vi "Configure CAN Read Gen.vi"(8 "error in":errorcluster, 11 "measurement configuration":T1 {"Baudrate" format="%x"; "FD Baudrate" format="%x"}) -> (0 "error out":errorcluster, 3 "XNET Read":refnum<k21>)   [LabVIEW 2025]
uses:
  <resource>/objmgr/xnet.rc
  <vilib>/xnet/xnet.llb/XNET Create Session (Frame Input Stream).vi
  can-lin/CAN-LIN Raw Bus Capture UI/Toggle.ctl
  can-lin/CAN-LIN Raw Bus Capture/Measurement Configuration.ctl
  can-lin/CAN-LIN Raw Bus Capture/CAN-LIN Raw Bus Capture.lvclass
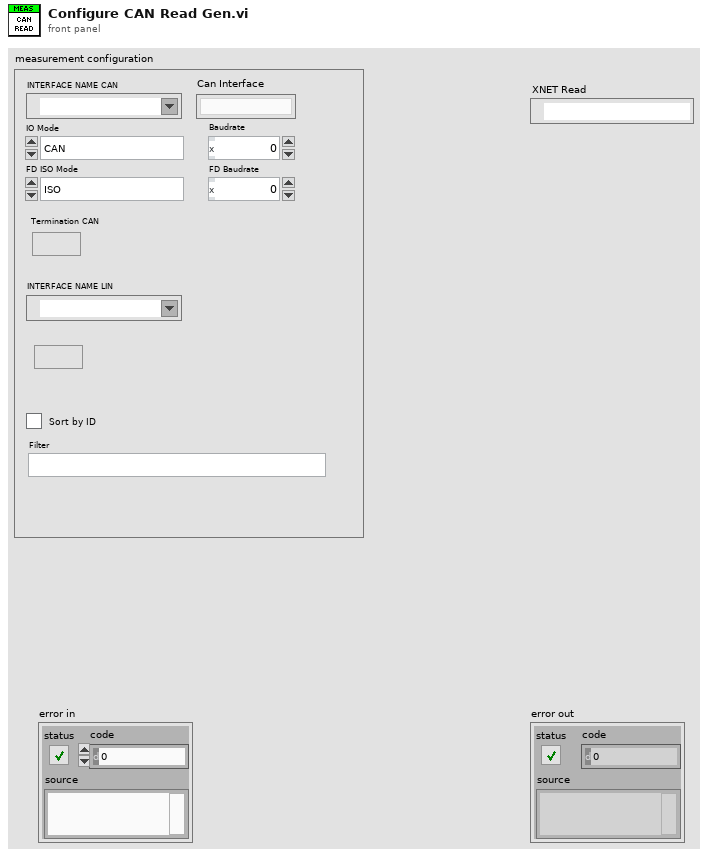
[diagram p1: front panel]
types:
  T1 = typedef "CAN-LIN Raw Bus Capture.lvclass/Measurement Configuration.ctl" = cluster{"INTERFACE NAME CAN":refnum<k21>, "Termination CAN":T2, "FD Baudrate":u32, "Baudrate":u32, "FD ISO Mode":enum32{"ISO", "Legacy ISO", "Non-ISO"}, "IO Mode":enum32{"CAN", "CAN FD", "CAN FD + BRS"}, "SortByID":bool, "Filter":string, "INTERFACE NAME LIN":refnum<k21>, "Termination LIN":T2, "Can Interface":string}
  T2 = typedef "Toggle.ctl" = bool
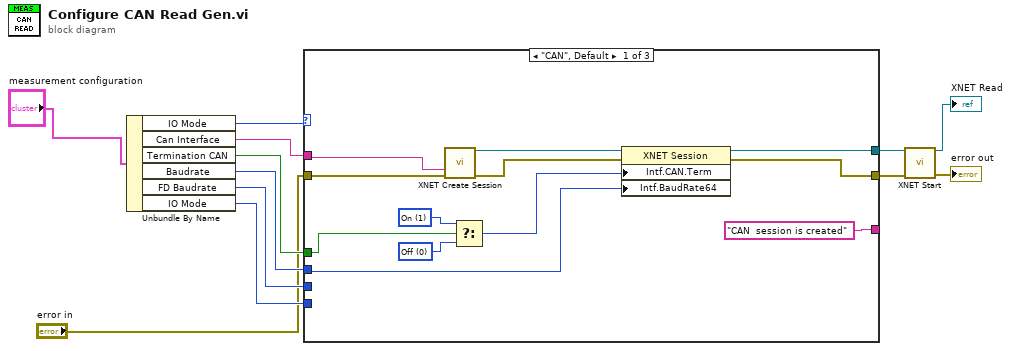
[diagram p0: block diagram]
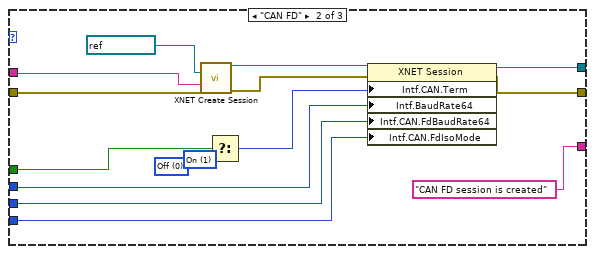
[diagram p2: hidden frame]
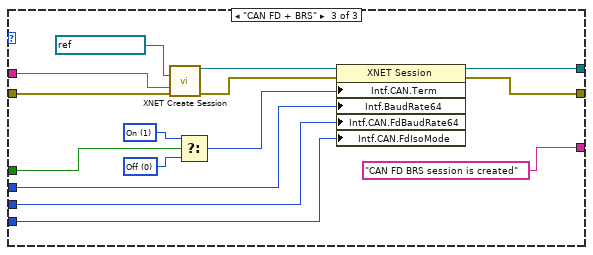
[diagram p3: hidden frame]
diagram:
  n1 = Unbundle By Name("measurement configuration") -> ("IO Mode"=w2:enum32{"CAN", "CAN FD", "CAN FD + BRS"}, "Can Interface"=w3:string, "Termination CAN"=w9:T2, "Baudrate"=w10:u32, "FD Baudrate"=w11:u32, "IO Mode"=w12:enum32{"CAN", "CAN FD", "CAN FD + BRS"})
  n2 = case shown="\"CAN\", Default" w2 {
    tunnel: [w19 w28 w48] -> w5
    tunnel: w3 -> [w14 w33 w43]
    tunnel: "error in" -> [w18 w32 w42]
    tunnel: [w17 w27 w41] -> w7
    tunnel: w9 -> [w16 w31 w47]
    tunnel: w10 -> [w15 w30 w46]
    tunnel: w11 -> [_ w26 w45]
    tunnel: w12 -> [_ w29 w44]
    tunnel: ["CAN  session is created" ("message") "CAN FD session is created" ("message") "CAN FD BRS session is created" ("message")] -> _
    frame "CAN", Default {
      w22 = u32 1 items=["Off", "On"] ("Interface:CAN:Termination")
      w21 = u32 0 items=["Off", "On"] ("Interface:CAN:Termination")
      n3 = call-poly <vilib>:"XNET Create Session.vi"("interface"=w14, "error in (no error)"=w18) -> ("session out"=w24:refnum<k21>, "error out"=w23:errorcluster)  [unwired: 12 in]
      n4 = Select(t=w22, s=w16, f=w21) -> (s? t:f=w20:u32)
      n5 = property class="XNET Session"(reference=w24, error in=w23, "Intf.CAN.Term"=w20, "Intf.BaudRate64"=w15) -> (reference out=w19:refnum<k21>, error out=w17:errorcluster)
    }
    frame "CAN FD" {
      w36 = u32 1 items=["Off", "On"] ("Interface:CAN:Termination")
      w35 = u32 0 items=["Off", "On"] ("Interface:CAN:Termination")
      n6 = call-poly <vilib>:"XNET Create Session.vi"("cluster (:memory:)"=refnum<k21> ":can_fd:", "interface"=w33, "error in (no error)"=w32) -> ("session out"=w38:refnum<k21>, "error out"=w37:errorcluster)  [unwired: 11 in]
      n7 = Select(t=w36, s=w31, f=w35) -> (s? t:f=w34:u32)
      n8 = property class="XNET Session"(reference=w38, error in=w37, "Intf.CAN.Term"=w34, "Intf.BaudRate64"=w30, "Intf.CAN.FdBaudRate64"=w26, "Intf.CAN.FdIsoMode"=w29) -> (reference out=w28:refnum<k21>, error out=w27:errorcluster)
    }
    frame "CAN FD + BRS" {
      w51 = u32 1 items=["Off", "On"] ("Interface:CAN:Termination")
      w50 = u32 0 items=["Off", "On"] ("Interface:CAN:Termination")
      n9 = call-poly <vilib>:"XNET Create Session.vi"("cluster (:memory:)"=refnum<k21> ":can_fd_brs:", "interface"=w43, "error in (no error)"=w42) -> ("session out"=w53:refnum<k21>, "error out"=w52:errorcluster)  [unwired: 11 in]
      n10 = Select(t=w51, s=w47, f=w50) -> (s? t:f=w49:u32)
      n11 = property class="XNET Session"(reference=w53, error in=w52, "Intf.CAN.Term"=w49, "Intf.BaudRate64"=w46, "Intf.CAN.FdBaudRate64"=w45, "Intf.CAN.FdIsoMode"=w44) -> (reference out=w48:refnum<k21>, error out=w41:errorcluster)
    }
  }
  n12 = call <vilib>:"XNET Start.vi"("session in"=w5, "error in (no error)"=w7) -> ("session out"=→"XNET Read":refnum<k21>, "error out"=→"error out":errorcluster)  [unwired: 12 in]
